vi "Popup Borders V2.vi"(10 "Row":cluster{"#":i16, "to #":i16}, 11 "VI refnum":refnum<vi>) -> ()   [LabVIEW 2012]
uses:
  Controls/Cell Border.ctl
  Controls/Row Borders [ ] Datas.ctl
panel:
  out "Array":string[](array[string])
  out "appended array":i16[](array[numeric])
  in  "Datas Row Borders [ ]":T1
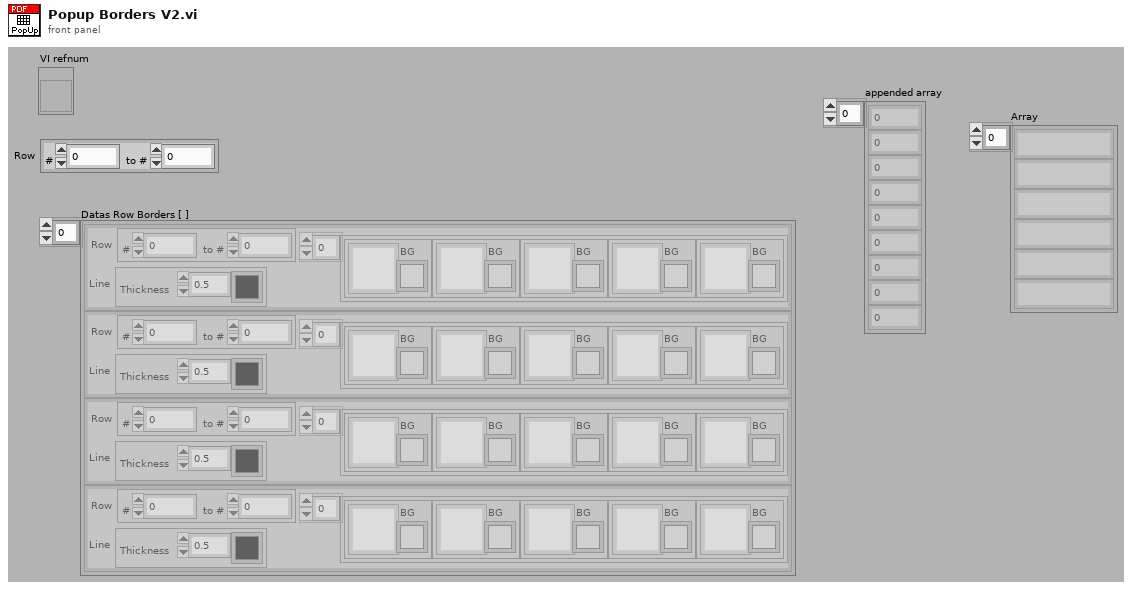
[diagram p1: front panel]
types:
  T1 = typedef "Row Borders [ ] Datas.ctl" = cluster{"Row":cluster{"#":i16, "to #":i16}, "Line":cluster{"Thickness":sgl, "Color":u32}, "Column Borders [ ]":cluster{"Cell Border":T2, "BG":u32}[]}[]
  T2 = typedef "Cell Border.ctl" = u16
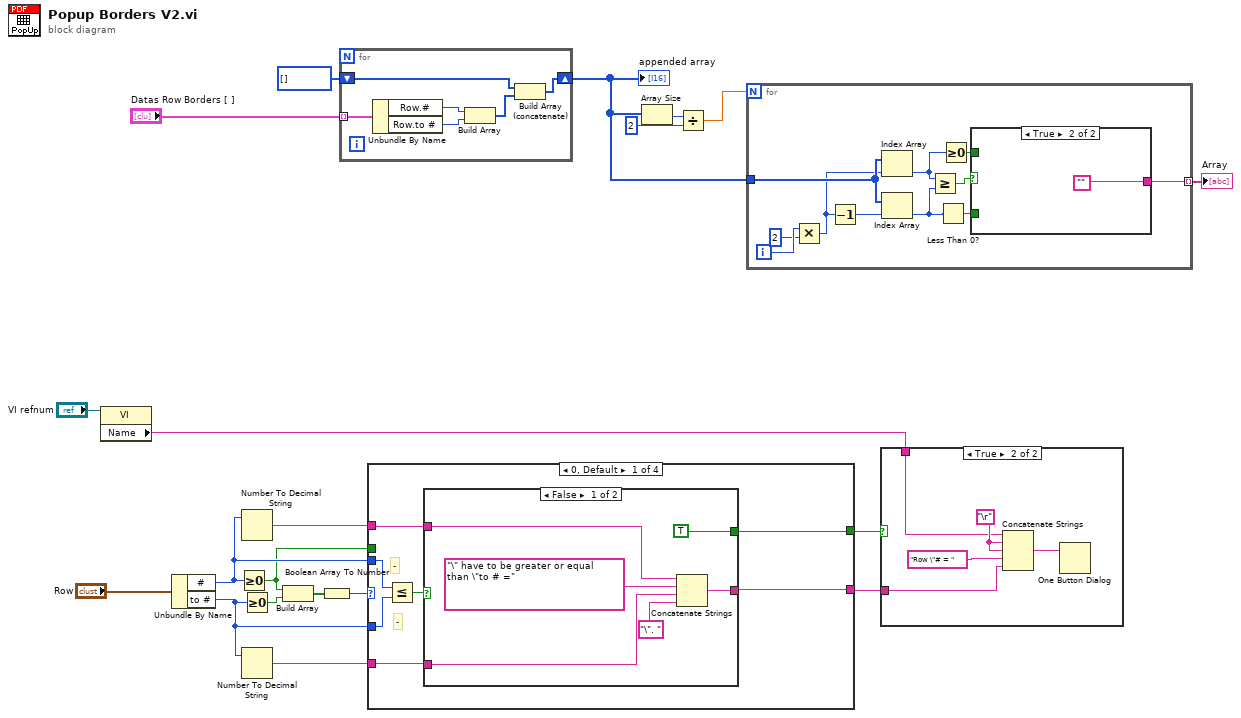
[diagram p0: block diagram]
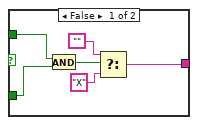
[diagram p2: hidden frame]
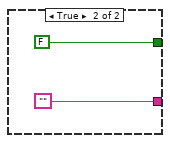
[diagram p3: hidden frame]
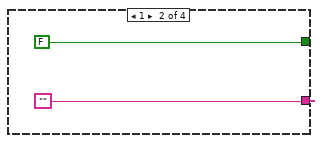
[diagram p4: hidden frame]
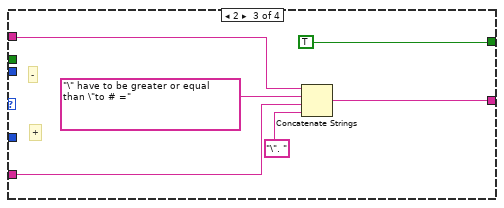
[diagram p5: hidden frame]
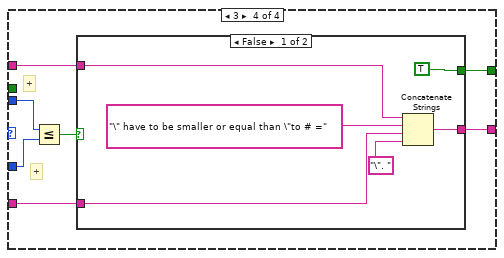
[diagram p6: hidden frame]
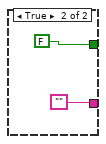
[diagram p7: hidden frame]
diagram:
  n1 = property class="VI"(reference="VI refnum") -> ("Name"=w20:string)  [unwired: 1 in, 2 out]
  n2 = Unbundle By Name("Row") -> ("#"=w15:i16, "to #"=w14:i16)
  n3 = Greater Or Equal To 0?(x=w15) -> (x >= 0?=w11:bool)
  n4 = Number To Decimal String(number=w15) -> (decimal integer string=w13:string)  [unwired: 1 out]
  n5 = Greater Or Equal To 0?(x=w14) -> (x >= 0?=w17:bool)
  n6 = Number To Decimal String(number=w14) -> (decimal integer string=w12:string)  [unwired: 1 out]
  n7 = Build Array(w11, w17) -> (w18:bool[])
  n8 = Boolean Array To Number(Boolean array=w18) -> (number=w16:u32)
  n9 = for {
    tunnel: "Datas Row Borders [ ]" -> [w26] mode=indexing
    shift-right: [w23] -> w2
    shift-left: i16[] [] ("appended array") -> [w22]
    n10 = Unbundle By Name(w26) -> ("Row.#"=w25:i16, "Row.to #"=w24:i16)
    n11 = Build Array(w25, w24) -> (w21:i16[])
    n12 = Build Array (concatenate)(w22, w21) -> (w23:i16[])
  }
  "appended array" <- w2
  n13 = case shown="0, Default" w16 {
    tunnel: w15 -> [w32 _ _ w55]
    tunnel: w14 -> [w33 _ _ w56]
    tunnel: w13 -> [w31 _ w49 w53]
    tunnel: w12 -> [w30 _ w48 w52]
    tunnel: [w28 FALSE TRUE w51] -> w10
    tunnel: [w27 "" w46 w50] -> w9
    tunnel: w11 -> [_ _ _ _]
    frame 0, Default {
      # "-"
      # "-"
      n14 = Less Or Equal?(x=w32, y=w33) -> (x <= y?=w29:bool)
      n15 = case shown="False" w29 {
        tunnel: [TRUE FALSE] -> w28
        tunnel: [w35 ""] -> w27
        tunnel: w31 -> [w37 _]
        tunnel: w30 -> [w36 _]
        frame False {
          n16 = Concatenate Strings(w37, "\" have to be greater or equal than \"to # =", w36, "\". ") -> (w35:string)
        }
        frame True {
        }
      }
    }
    frame 1 {
    }
    frame 2 {
      # "+"
      # "-"
      n17 = Concatenate Strings(w49, "\" have to be greater or equal than \"to # =", w48, "\". ") -> (w46:string)
    }
    frame 3 {
      # "+"
      # "+"
      n18 = Less Or Equal?(x=w55, y=w56) -> (x <= y?=w54:bool)
      n19 = case shown="False" w54 {
        tunnel: [TRUE FALSE] -> w51
        tunnel: w53 -> [w60 _]
        tunnel: w52 -> [w59 _]
        tunnel: [w58 ""] -> w50
        frame False {
          n20 = Concatenate Strings(w60, "\" have to be smaller or equal than \"to # =", w59, "\". ") -> (w58:string)
        }
        frame True {
        }
      }
    }
  }
  n21 = Array Size(array=w2) -> (size(s)=w5:i32)
  n22 = Divide(x=w5, y=2) -> (x/y=w3:dbl)
  n23 = for {
    N: w3 -> [_]
    tunnel: w2 -> [w73]
    tunnel: [w65] -> w1 mode=indexing
    i -> [w75]
    n24 = Multiply(x=w75, y=2) -> (x*y=w72:i32)
    n25 = Decrement(x=w72) -> (x-1=w71:i32)
    n26 = Index Array(array=w73, index=w72) -> (element=w68:i16)
    n27 = Index Array(array=w73, index=w71) -> (element=w69:i16)
    n28 = Greater Or Equal?(x=w68, y=w69) -> (x >= y?=w70:bool)
    n29 = Less Than 0?(x=w69) -> (x < 0?=w66:bool)
    n30 = Greater Or Equal To 0?(x=w68) -> (x >= 0?=w67:bool)
    n31 = case shown="True" w70 {
      tunnel: w67 -> [w81 _]
      tunnel: w66 -> [w80 _]
      tunnel: [w77 ""] -> w65
      frame False {
        n32 = And(x=w81, y=w80) -> (x .and. y?=w79:bool)
        n33 = Select(t="", s=w79, f="X") -> (s? t:f=w77:string)
      }
      frame True {
      }
    }
  }
  "Array" <- w1
  n34 = case shown="True" w10 {
    tunnel: w20 -> [_ w85]
    tunnel: w9 -> [_ w83]
    frame False {
    }
    frame True {
      w86 = "\r"
      n35 = Concatenate Strings(w85, w86, w86, "Row \"# = ", w83) -> (w87:string)
      n36 = One Button Dialog(message=w87) -> ()  [unwired: 2 out]
    }
  }
